vi "Increment_Variables_accel.vi"(0 "Accelerometer":waveform(dbl)[](array[waveform])=[{"t0"=timestamp(3695932468.9735494 s since 1904-01-01), "dt"=0.001015625, "Y"=[0.019294717668341704, 0.03864380419095477, -0.011709081788944725, -0.0416190732361809, -0.043655819185929645, -0.029323162502512563, 0.0026990099296482425, 0.0025104223417085417, -0.030530123065326632, -0.014575613125628141, 0.030044210180904515, 0.011411756492462309, 0.011675779115577892, 0.05037395216080402, 0.03887010929648241, 0.022802446804020104, -0.013368652562814068, -0.05123704022110553, -0.041053310472361805, -0.03415100475376884, -0.020120088211055275, 0.015221225768844215, 0.03291074151758794, 0.0006622639798994981, -0.04222255351758794, -0.05044497235175879, -0.047616158532663315, -0.03682894850251256, -0.026041738472361808, -0.006768086984924621, 0.0323072612361809, 0.03094943060301507, -0.006730369467336683, -0.035735140492462306, -0.017668449567839195, 0.016352751296482407, -0.005259386281407034, -0.021477918844221105, 0.014504592934673363, 0.056635060080402005, 0.050072212020100496, 0.04184979318592964, 0.019143847597989955, -0.009257443145728642, 0.02483919275376885, 0.0027744449648241173, 0.0039059704924623087, 0.03128888826130653, 0.0039059704924623087, 0.03498520498492462, 0.053579941155778896, 0.0218595088643216, 0.006923371899497488, 0.039511307095477385, 0.054334291507537685, 0.03419313711557789, 0.010996863798994977, -0.034226439788944726, -0.033094914261306535, -0.014651048160804023, 0.014165135276381913, 0.05599386228140703, 0.046300460261306534, 0.02921442479396985, -0.001638504592964822, -0.03852623679396985, -0.017479861979899494, 0.008620660190954775, -0.010464403708542715, -0.03618775070351758, -0.001336764452261309, 0.025442673035175875, -0.013481805115577887, 0.009450445577889446, 0.007753157286432159, -0.018007907226130652, 0.011223168904522615, -0.028908269809045224, -0.03950689225125628, -0.013180064974874374, 0.0145423104522613, 0.06338649572864322, 0.05252385066331658, 0.04656448288442211, 0.022576141698492466, -0.003147205296482415, 0.03698423341708543, 0.03860608667336683, -0.0006955666532663315, -0.022383139266331658, -0.0009595892763819072, 0.0520712404522613, 0.05931300382914573, 0.04928014415075377, 0.0396244596482412, 0.005112931055276382, 0.03434400718592964, 0.06602672195979899, 0.05060025726633166, 0.04909155656281407, 0.015070355698492466, 0.021482333688442212, 0.06904412336683417, 0.07209924229145728, 0.07074141165829145, 0.0710808693165829, 0.06851607812060301, 0.06723368252261307, 0.06557411174874371, 0.06157605488442211, 0.06199094757788945, 0.05633331993969849, 0.05210895796984924, 0.032873024, 0.008545225155778893, 0.04645133033165828, 0.06832749053266331, 0.05671049511557788, 0.05407026888442211, 0.04415056175879396, 0.015522965909547742, 0.007790874804020097, 0.05033623464321607, 0.052372980592964816, 0.032873024, 0.012203824361809043, -0.02445760273366834, -0.006692651949748746, 0.04177435815075377, 0.06640389713567839, 0.062179535165829136, 0.049883624432160795, 0.04286816616080402, 0.012694152090452257, -0.004844493587939695, 0.027932029195979896, 0.030232797768844216, -0.01687638169849246, -0.03818677913567839, -0.031322190934673366, -0.005561126422110554, 0.028384639407035173, 0.04520665225125628, 0.014881768110552765, -0.012689737246231153, 0.02189722638190955, -0.0015630695577889472, -0.004014708201005024, 0.01940787022110553, -0.01815877729648241, 0.009035552884422107, -0.0007710016884422133, -0.03158621355778894, 0.015786988532663318, 0.05365537619095477, 0.06059539942713567, 0.05033623464321607, 0.03977532971859296, 0.015862423567839193, -0.026192608542713568, -0.04233570607035175, -0.008616245346733671, -0.003034052743718596, -0.04576800017085427, -0.05161421539698492, -0.03550883538693467, -0.0341132872361809, 0.0026990099296482425, 0.026159305869346727, -0.0029586177085427143, 0.02246298914572864, 0.039322719507537685, -0.0004315440301507559, -0.03350980695477387, -0.033962417165829144, 0.003943688010050253, -0.013481805115577887, -0.0423734235879397, -0.03147306100502512, -0.009031138040201003, 0.03438172470351758, 0.05071340981909547, 0.025329520482412063, 0.001944659577889446, 0.04207609829145728, 0.05886039361809045, 0.041208595386934666, 0.03215639116582915, -0.007711024924623118, 0.020463960713567833, 0.025103215376884425, 0.006810219346733669, 0.05440972654271356, 0.06383910593969849, 0.055164076894472364, 0.04645133033165828, 0.03155291088442211, -0.006579499396984927, 0.0013788968140703503, 0.0176728644120603], "attributes"=variant("NI_ChannelName"=variant(string "cDAQ2Mod4/ai0"), "NI_UnitDescription"=variant(string "g"), "NI_dBReference"=variant(dbl 1.0))}, {"t0"=timestamp(3695932468.9735494 s since 1904-01-01), "dt"=0.001015625, "Y"=[0.009095719096509247, 0.02787151909650923, -0.02309687433264887, -0.05374730759753593, -0.056099101848049275, -0.04040762217659137, -0.008176474743326487, -0.00914032484599589, -0.04256664640657083, -0.027376368788501027, 0.019004098151950727, 0.0018475663244353208, 0.0016547963039014318, 0.04047867843942504, 0.026869114989733045, 0.010560771252566742, -0.024022170431211493, -0.06300026858316221, -0.05374730759753593, -0.045882290759753586, -0.03138598521560575, 0.003351172484599582, 0.02247395852156056, -0.010065620944558526, -0.0547497117043121, -0.06219063449691991, -0.05976173223819301, -0.04842685503080081, -0.03701486981519507, -0.01715955770020533, 0.022512512525667355, 0.020353488295687894, -0.016311369609856255, -0.04800276098562628, -0.02957394702258727, 0.006242722792607805, -0.018200515811088294, -0.03312091540041068, 0.003929482546201235, 0.04599190102669404, 0.039322058316221764, 0.03145704147843942, 0.007784882956878847, -0.02244145626283367, 0.014377617659137587, -0.007945150718685831, -0.0068656386036961, 0.02201131047227925, -0.006672868583162211, 0.024671536755646817, 0.04390998480492814, 0.012257147433264892, -0.004436736344969203, 0.029413679260780284, 0.04514371293634495, 0.02181854045174539, -0.00011868788501026573, -0.045419642710472274, -0.04511121067761806, -0.025911316632443532, 0.002040336344969196, 0.04595334702258727, 0.03673894004106776, 0.01861855811088295, -0.011723443121149896, -0.05023889322381929, -0.028532988911704305, -0.001429524024640652, -0.021747484188911703, -0.047617220944558517, -0.013458373305954827, 0.015418575770020537, -0.022749888295687887, -0.002393374127310055, -0.00451384435318275, -0.030267919096509235, -0.0005427819301848102, -0.039597988090349076, -0.05139551334702258, -0.025641438603696096, 0.003968036550308002, 0.0528545137577002, 0.04221360862422996, 0.0366618320328542, 0.011254743326488709, -0.014383669404517449, 0.027061885010266934, 0.028218505133470212, -0.012455969199178643, -0.03439319753593428, -0.01253307720739219, 0.04094132648870635, 0.04822803326488706, 0.03909073429158111, 0.029336571252566723, -0.005400586447638606, 0.024247442710472272, 0.05636292813141683, 0.04117265051334701, 0.03793411416837783, 0.004160806570841891, 0.011678837371663253, 0.059331586447638585, 0.06280144681724845, 0.061683380698151935, 0.061490610677618074, 0.058560506365503084, 0.05805930431211498, 0.05613160410677617, 0.051967771663244344, 0.05273885174537987, 0.04664731909650924, 0.04175096057494865, 0.022512512525667355, -0.0014680780287474327, 0.036199183983572886, 0.05925447843942505, 0.04830514127310062, 0.04417986283367556, 0.03307630965092401, 0.005008994661190966, -0.0022777121149897273, 0.03982326036960984, 0.04325456673511294, 0.023360700616016417, 0.0010764862422997928, -0.03578114168377823, -0.018547501848049278, 0.03126427145790553, 0.056594252156057484, 0.051389461601642705, 0.038936518275153986, 0.03323052566735113, 0.0014620262833675568, -0.017082449691991783, 0.019004098151950727, 0.020353488295687894, -0.027222152772073918, -0.0486196250513347, -0.04333772648870636, -0.016311369609856255, 0.018155910061601638, 0.035081117864476374, 0.003351172484599582, -0.024484818480492804, 0.011563175359342925, -0.012417415195071863, -0.014576439425051338, 0.008864395071868592, -0.02891852895277207, -0.0011981999999999965, -0.010952363039014368, -0.04179556632443532, 0.004623454620123202, 0.044218416837782326, 0.05250752772073922, 0.03966904435318275, 0.028719707186858318, 0.004315022587268999, -0.03759317987679671, -0.05316899753593428, -0.020012554004106772, -0.014268007392197121, -0.059800286242299786, -0.06488941478439425, -0.0461907227926078, -0.045419642710472274, -0.007212624640657084, 0.016652303901437376, -0.014113791375770013, 0.010830649281314164, 0.029220909240246395, -0.011260795071868585, -0.04507265667351129, -0.044802778644763855, -0.007945150718685831, -0.02413783244353182, -0.054055739630390134, -0.044648562628336746, -0.019742675975359336, 0.024864306776180706, 0.04229071663244352, 0.016305317864476393, -0.008060812731006159, 0.03191968952772073, 0.047341291170431204, 0.031302825462012324, 0.02247395852156056, -0.01904870390143737, 0.011177635318275148, 0.016305317864476393, -0.003241562217659144, 0.04452684887063654, 0.05485932197125257, 0.04595334702258727, 0.0365076160164271, 0.02181854045174539, -0.018046299794661186, -0.009988512936344965, 0.006088506776180697], "attributes"=variant("NI_ChannelName"=variant(string "cDAQ2Mod4/ai1"), "NI_UnitDescription"=variant(string "g"), "NI_dBReference"=variant(dbl 1.0))}, {"t0"=timestamp(3695932468.9735494 s since 1904-01-01), "dt"=0.001015625, "Y"=[0.02589708890303623, 0.04288576104799216, -0.00554298617042116, -0.03396775579823702, -0.036210848873653285, -0.02234779822722821, 0.008871644740450536, 0.008540696581782563, -0.023598046826640552, -0.00903632784524976, 0.035237181380999016, 0.01777047300685602, 0.017035032654260523, 0.05546179107737512, 0.04402569359451518, 0.02814018197845249, -0.005469442135161609, -0.04308721617042116, -0.03374712369245837, -0.02554696376101861, -0.013265109872673852, 0.02001356608227228, 0.038767295073457386, 0.008099432370225267, -0.034298703956905, -0.04367556845249755, -0.04091766713026445, -0.029408025612144957, -0.017898384094025468, 0.0018481893731635626, 0.03832603086190009, 0.03670806208619, 0.0012230650734573918, -0.029628657717923605, -0.011683913114593538, 0.022808239422135158, 0.0007450288442703186, -0.013963778207639572, 0.019682617923604307, 0.06009506529872673, 0.054946982830558266, 0.04637910272282075, 0.02299209951028403, -0.004954633888344762, 0.030898083300685598, 0.008834872722820759, 0.009202592899118508, 0.03648742998041135, 0.009717401145935351, 0.04016463174338883, 0.05689589976493632, 0.027404741625856998, 0.01302688273261508, 0.04520239815866796, 0.06009506529872673, 0.03784799463271302, 0.016667312477962774, -0.027091388501469152, -0.027091388501469152, -0.008227343457394714, 0.019204581694417234, 0.060646645563173354, 0.05167427326150831, 0.03468560111655239, 0.005856339294809009, -0.03098922237022527, -0.010727840656219395, 0.015159659755142014, -0.003998561429970619, -0.02870935727717924, 0.003429386131243873, 0.030567135142017626, -0.005726846258570034, 0.014718395543584718, 0.01302688273261508, -0.011794229167482862, 0.01637313633692458, -0.02227425419196866, -0.032386559040156714, -0.0074551310871694455, 0.019903250029382955, 0.06719206470127324, 0.05605014335945151, 0.05185813334965719, 0.028066637943192942, 0.0031719820078354513, 0.043437341312438774, 0.04317993718903035, 0.004091282448579821, -0.016243643300685603, 0.004348686571988242, 0.05538824704211556, 0.0630368267091087, 0.054064454407443674, 0.04428309771792359, 0.012364986415279135, 0.0403484918315377, 0.06994996602350635, 0.055866283271302636, 0.052740661772771785, 0.020932866523016642, 0.027625373731635646, 0.07399488796278157, 0.07822366999020566, 0.07495096042115572, 0.07590703287952986, 0.07333299164544563, 0.07248723523996081, 0.07112667058765915, 0.06579472803134181, 0.06612567619000978, 0.05958025705190988, 0.056270775465230155, 0.03884083910871694, 0.01519643177277179, 0.05075497282076395, 0.07322267559255631, 0.06307359872673848, 0.05814614836434867, 0.04917377606268364, 0.02148444678746327, 0.013799095102840348, 0.05590305528893241, 0.058109376346718894, 0.03946596340842311, 0.018653001429970614, -0.017346803829578848, -0.0006523078256611206, 0.047776439392752196, 0.07112667058765915, 0.06550055189030361, 0.05520438695396669, 0.048879599921645436, 0.01857945739471106, 0.0004140806856023464, 0.0333618084818805, 0.03630356989226248, -0.010360120479921648, -0.0313937145641528, -0.025399875690499514, 0.00045085270323211996, 0.034354652957884424, 0.051122692997061694, 0.022109571087169436, -0.005212038011753187, 0.028912394348677758, 0.005157670959843288, 0.002179137531831535, 0.02611772100881488, -0.011426508991185115, 0.015821556072477958, 0.0065550076297747235, -0.024076083055827622, 0.02291855547502448, 0.05950671301665034, 0.06605213215475024, 0.05472635072477962, 0.04428309771792359, 0.021337358716944168, -0.019038316640548485, -0.033820667727717926, -0.002490908707149856, 0.003907422360430946, -0.039704190548481885, -0.04632315372184133, -0.027532652713026448, -0.026797212360430953, 0.010158665357492647, 0.03225864795298726, 0.0012598370910871654, 0.02791954987267384, 0.04608492658178255, 0.006260831488736528, -0.026208860078354556, -0.025877911919686584, 0.01048961351616062, -0.005763618276199808, -0.03451933606268365, -0.023303870685602354, -0.0006890798432908941, 0.0388776111263467, 0.05616045941234084, 0.03317794839373163, 0.008540696581782563, 0.04593783851126346, 0.06255879047992163, 0.047371947198824677, 0.037553818491674815, -0.0025644527424094066, 0.0275518296963761, 0.03266314014691478, 0.013247514838393728, 0.06002152126346717, 0.06936161374142996, 0.06009506529872673, 0.05193167738491673, 0.037480274456415275, -2.71835259549498e-05, 0.007694940176297741, 0.022661151351616057], "attributes"=variant("NI_ChannelName"=variant(string "cDAQ2Mod4/ai2"), "NI_UnitDescription"=variant(string "g"), "NI_dBReference"=variant(dbl 1.0))}], 7 "Dummy Variable":dbl, 11 "error in 2":errorcluster) -> (1 "Y Accel Mag Array":dbl[](array[numeric])=[0.0033131967905544145, 0.011533831525713547, 0.008442061667059993, 0.009858654673222715, 0.008363300405539103, 0.002102550987145263, 0.004096487024183529, 0.00433165841994114, 0.00265508252937339, 0.005003543741433319, 0.0033674389332133095, 0.002412892363694339, 0.0017371897457633865, 0.0017333218339316864, 0.005254413350826224, 0.0073063809360835764, 0.00608380643471068, 0.0054542062991900335, 0.0023792094373612746, 0.004789200183006362, 0.007375237173938309, 0.003195183497815143, 0.0023576659519010824, 0.0031894685751027315, 0.0038472288041279876, 0.00184315376000046, 0.0050331931255288365, 0.0037747131768431563, 0.0014627035558359514, 0.003750056064901884, 0.005614898068157985, 0.005092169153670107, 0.006887608554409304, 0.0030983879127384735, 0.00214165531724511, 0.0003241083331647927, 0.0007980815831222994, 0.0035613760739590596, 0.00390793128896121, 0.003400370462350215, 0.004733205931244773, 0.003908201318260342, 0.000856924466573951, 0.0020338139877837543, 0.0026238508086522004, 0.000830066713475989, 0.0038902184256169644, 0.0031358154993883698, 0.0008589993939411568, 0.002873307167999069, 0.0023416434646463687, 0.0004510931593907119, 0.0004383783165562844, 0.0008874627311727322, 0.0012789681306284875, 0.0002755434129271385, 0.001522428187930964, 0.0025118502280273036, 0.0010763668998756048, 0.0017983248042534833, 0.0005603708597797223, 0.002488708057422721, 0.0034289499116928156, 0.0005141761317015294, 0.0005662749543606555, 0.0005895376750470246, 0.001316995707438423, 0.0019666607616864824, 0.0008909162596128791, 0.0018501545019689312, 0.0033674680981186198, 0.0018638646097661321, 0.0009231644052021042, 0.0013305685669963152, 0.00048467212646142815, 0.0010055563426380114, 0.0011922512362583773, 0.0013757679345206871, 0.001722787838392562, 0.001379941884811358, 0.0003961471539844812, 0.0017666790214067446, 0.0006913734583918143, 0.00154018788064677, 0.0010101793664572742, 0.00042212007045419495, 0.0006835355378316494, 0.001188644910899636, 0.00040022276319623824, 6.267596269438565e-05, 0.00011130714088648695, 0.00029044914834298766, 0.00013994679469761935, 9.599722391194053e-05, 0.00011490038035474606, 8.073681312813299e-05, 6.818183165259488e-05, 5.3847083164786216e-05, 4.243495671007987e-05, 3.670183062517156e-05], 3 "Y Accel Freq Array":dbl[](array[numeric])=[0.0, 4.923076923076923, 9.846153846153847, 14.76923076923077, 19.692307692307693, 24.615384615384617, 29.53846153846154, 34.46153846153847, 39.38461538461539, 44.30769230769231, 49.230769230769226, 54.153846153846146, 59.076923076923066, 63.999999999999986, 68.9230769230769, 73.84615384615383, 78.76923076923075, 83.69230769230766, 88.61538461538458, 93.5384615384615, 98.46153846153842, 103.38461538461534, 108.30769230769226, 113.23076923076918, 118.1538461538461, 123.07692307692302, 127.99999999999994, 132.92307692307688, 137.8461538461538, 142.76923076923075, 147.69230769230768, 152.6153846153846, 157.53846153846155, 162.46153846153848, 167.38461538461542, 172.30769230769235, 177.23076923076928, 182.15384615384622, 187.07692307692315, 192.00000000000009, 196.92307692307702, 201.84615384615395, 206.7692307692309, 211.69230769230782, 216.61538461538476, 221.5384615384617, 226.46153846153862, 231.38461538461556, 236.3076923076925, 241.23076923076943, 246.15384615384636, 251.0769230769233, 256.0000000000002, 260.92307692307713, 265.84615384615404, 270.76923076923094, 275.69230769230785, 280.61538461538476, 285.53846153846166, 290.46153846153857, 295.3846153846155, 300.3076923076924, 305.2307692307693, 310.1538461538462, 315.0769230769231, 320.0, 324.9230769230769, 329.8461538461538, 334.7692307692307, 339.6923076923076, 344.6153846153845, 349.53846153846143, 354.46153846153834, 359.38461538461524, 364.30769230769215, 369.23076923076906, 374.15384615384596, 379.07692307692287, 383.9999999999998, 388.9230769230767, 393.8461538461536, 398.7692307692305, 403.6923076923074, 408.6153846153843, 413.5384615384612, 418.4615384615381, 423.384615384615, 428.3076923076919, 433.23076923076883, 438.15384615384573, 443.07692307692264, 447.99999999999955, 452.92307692307645, 457.84615384615336, 462.76923076923026, 467.69230769230717, 472.6153846153841, 477.538461538461, 482.4615384615379, 487.3846153846148, 492.3076923076917, 497.2307692307686], 4 "Time Stamp":timestamp[](array[timestamp])=[timestamp(3695932468.9735494 s since 1904-01-01), timestamp(3695932468.974565 s since 1904-01-01), timestamp(3695932468.9755807 s since 1904-01-01), timestamp(3695932468.9765964 s since 1904-01-01), timestamp(3695932468.977612 s since 1904-01-01), timestamp(3695932468.9786277 s since 1904-01-01), timestamp(3695932468.9796433 s since 1904-01-01), timestamp(3695932468.980659 s since 1904-01-01), timestamp(3695932468.981674 s since 1904-01-01), timestamp(3695932468.98269 s since 1904-01-01), timestamp(3695932468.9837055 s since 1904-01-01), timestamp(3695932468.984721 s since 1904-01-01), timestamp(3695932468.985737 s since 1904-01-01), timestamp(3695932468.9867525 s since 1904-01-01), timestamp(3695932468.987768 s since 1904-01-01), timestamp(3695932468.988784 s since 1904-01-01), timestamp(3695932468.9897995 s since 1904-01-01), timestamp(3695932468.990815 s since 1904-01-01), timestamp(3695932468.991831 s since 1904-01-01), timestamp(3695932468.9928465 s since 1904-01-01), timestamp(3695932468.993862 s since 1904-01-01), timestamp(3695932468.9948773 s since 1904-01-01), timestamp(3695932468.995893 s since 1904-01-01), timestamp(3695932468.9969087 s since 1904-01-01), timestamp(3695932468.9979243 s since 1904-01-01), timestamp(3695932468.99894 s since 1904-01-01), timestamp(3695932468.9999557 s since 1904-01-01), timestamp(3695932469.0009713 s since 1904-01-01), timestamp(3695932469.001987 s since 1904-01-01), timestamp(3695932469.0030026 s since 1904-01-01), timestamp(3695932469.0040183 s since 1904-01-01), timestamp(3695932469.005034 s since 1904-01-01), timestamp(3695932469.0060496 s since 1904-01-01), timestamp(3695932469.007065 s since 1904-01-01), timestamp(3695932469.0080805 s since 1904-01-01), timestamp(3695932469.009096 s since 1904-01-01), timestamp(3695932469.010112 s since 1904-01-01), timestamp(3695932469.0111275 s since 1904-01-01), timestamp(3695932469.012143 s since 1904-01-01), timestamp(3695932469.013159 s since 1904-01-01), timestamp(3695932469.0141745 s since 1904-01-01), timestamp(3695932469.01519 s since 1904-01-01), timestamp(3695932469.016206 s since 1904-01-01), timestamp(3695932469.0172215 s since 1904-01-01), timestamp(3695932469.018237 s since 1904-01-01), timestamp(3695932469.019253 s since 1904-01-01), timestamp(3695932469.020268 s since 1904-01-01), timestamp(3695932469.0212836 s since 1904-01-01), timestamp(3695932469.0222993 s since 1904-01-01), timestamp(3695932469.023315 s since 1904-01-01), timestamp(3695932469.0243306 s since 1904-01-01), timestamp(3695932469.0253463 s since 1904-01-01), timestamp(3695932469.026362 s since 1904-01-01), timestamp(3695932469.0273776 s since 1904-01-01), timestamp(3695932469.0283933 s since 1904-01-01), timestamp(3695932469.029409 s since 1904-01-01), timestamp(3695932469.0304246 s since 1904-01-01), timestamp(3695932469.0314403 s since 1904-01-01), timestamp(3695932469.0324554 s since 1904-01-01), timestamp(3695932469.033471 s since 1904-01-01), timestamp(3695932469.034487 s since 1904-01-01), timestamp(3695932469.0355024 s since 1904-01-01), timestamp(3695932469.036518 s since 1904-01-01), timestamp(3695932469.0375338 s since 1904-01-01), timestamp(3695932469.0385494 s since 1904-01-01), timestamp(3695932469.039565 s since 1904-01-01), timestamp(3695932469.0405807 s since 1904-01-01), timestamp(3695932469.0415964 s since 1904-01-01), timestamp(3695932469.042612 s since 1904-01-01), timestamp(3695932469.0436277 s since 1904-01-01), timestamp(3695932469.0446434 s since 1904-01-01), timestamp(3695932469.0456586 s since 1904-01-01), timestamp(3695932469.0466743 s since 1904-01-01), timestamp(3695932469.04769 s since 1904-01-01), timestamp(3695932469.0487056 s since 1904-01-01), timestamp(3695932469.0497212 s since 1904-01-01), timestamp(3695932469.050737 s since 1904-01-01), timestamp(3695932469.0517526 s since 1904-01-01), timestamp(3695932469.052768 s since 1904-01-01), timestamp(3695932469.053784 s since 1904-01-01), timestamp(3695932469.0547996 s since 1904-01-01), timestamp(3695932469.055815 s since 1904-01-01), timestamp(3695932469.056831 s since 1904-01-01), timestamp(3695932469.057846 s since 1904-01-01), timestamp(3695932469.0588617 s since 1904-01-01), timestamp(3695932469.0598774 s since 1904-01-01), timestamp(3695932469.060893 s since 1904-01-01), timestamp(3695932469.0619087 s since 1904-01-01), timestamp(3695932469.0629244 s since 1904-01-01), timestamp(3695932469.06394 s since 1904-01-01), timestamp(3695932469.0649557 s since 1904-01-01), timestamp(3695932469.0659714 s since 1904-01-01), timestamp(3695932469.066987 s since 1904-01-01), timestamp(3695932469.0680027 s since 1904-01-01), timestamp(3695932469.0690184 s since 1904-01-01), timestamp(3695932469.070034 s since 1904-01-01), timestamp(3695932469.071049 s since 1904-01-01), timestamp(3695932469.072065 s since 1904-01-01), timestamp(3695932469.0730805 s since 1904-01-01), timestamp(3695932469.074096 s since 1904-01-01), timestamp(3695932469.075112 s since 1904-01-01), timestamp(3695932469.0761275 s since 1904-01-01), timestamp(3695932469.077143 s since 1904-01-01), timestamp(3695932469.078159 s since 1904-01-01), timestamp(3695932469.0791745 s since 1904-01-01), timestamp(3695932469.08019 s since 1904-01-01), timestamp(3695932469.081206 s since 1904-01-01), timestamp(3695932469.0822215 s since 1904-01-01), timestamp(3695932469.0832367 s since 1904-01-01), timestamp(3695932469.0842524 s since 1904-01-01), timestamp(3695932469.085268 s since 1904-01-01), timestamp(3695932469.0862837 s since 1904-01-01), timestamp(3695932469.0872993 s since 1904-01-01), timestamp(3695932469.088315 s since 1904-01-01), timestamp(3695932469.0893307 s since 1904-01-01), timestamp(3695932469.0903463 s since 1904-01-01), timestamp(3695932469.091362 s since 1904-01-01), timestamp(3695932469.0923777 s since 1904-01-01), timestamp(3695932469.0933933 s since 1904-01-01), timestamp(3695932469.094409 s since 1904-01-01), timestamp(3695932469.0954247 s since 1904-01-01), timestamp(3695932469.09644 s since 1904-01-01), timestamp(3695932469.0974555 s since 1904-01-01), timestamp(3695932469.098471 s since 1904-01-01), timestamp(3695932469.099487 s since 1904-01-01), timestamp(3695932469.1005025 s since 1904-01-01), timestamp(3695932469.101518 s since 1904-01-01), timestamp(3695932469.102534 s since 1904-01-01), timestamp(3695932469.1035495 s since 1904-01-01), timestamp(3695932469.104565 s since 1904-01-01), timestamp(3695932469.105581 s since 1904-01-01), timestamp(3695932469.1065965 s since 1904-01-01), timestamp(3695932469.107612 s since 1904-01-01), timestamp(3695932469.1086273 s since 1904-01-01), timestamp(3695932469.109643 s since 1904-01-01), timestamp(3695932469.1106586 s since 1904-01-01), timestamp(3695932469.1116743 s since 1904-01-01), timestamp(3695932469.11269 s since 1904-01-01), timestamp(3695932469.1137056 s since 1904-01-01), timestamp(3695932469.1147213 s since 1904-01-01), timestamp(3695932469.115737 s since 1904-01-01), timestamp(3695932469.1167526 s since 1904-01-01), timestamp(3695932469.1177683 s since 1904-01-01), timestamp(3695932469.118784 s since 1904-01-01), timestamp(3695932469.1197996 s since 1904-01-01), timestamp(3695932469.1208153 s since 1904-01-01), timestamp(3695932469.1218305 s since 1904-01-01), timestamp(3695932469.122846 s since 1904-01-01), timestamp(3695932469.123862 s since 1904-01-01), timestamp(3695932469.1248775 s since 1904-01-01), timestamp(3695932469.125893 s since 1904-01-01), timestamp(3695932469.126909 s since 1904-01-01), timestamp(3695932469.1279244 s since 1904-01-01), timestamp(3695932469.12894 s since 1904-01-01), timestamp(3695932469.129956 s since 1904-01-01), timestamp(3695932469.1309714 s since 1904-01-01), timestamp(3695932469.131987 s since 1904-01-01), timestamp(3695932469.1330028 s since 1904-01-01), timestamp(3695932469.134018 s since 1904-01-01), timestamp(3695932469.1350336 s since 1904-01-01), timestamp(3695932469.1360493 s since 1904-01-01), timestamp(3695932469.137065 s since 1904-01-01), timestamp(3695932469.1380806 s since 1904-01-01), timestamp(3695932469.1390963 s since 1904-01-01), timestamp(3695932469.140112 s since 1904-01-01), timestamp(3695932469.1411276 s since 1904-01-01), timestamp(3695932469.1421432 s since 1904-01-01), timestamp(3695932469.143159 s since 1904-01-01), timestamp(3695932469.1441746 s since 1904-01-01), timestamp(3695932469.1451902 s since 1904-01-01), timestamp(3695932469.146206 s since 1904-01-01), timestamp(3695932469.147221 s since 1904-01-01), timestamp(3695932469.1482368 s since 1904-01-01), timestamp(3695932469.1492524 s since 1904-01-01), timestamp(3695932469.150268 s since 1904-01-01), timestamp(3695932469.1512837 s since 1904-01-01), timestamp(3695932469.1522994 s since 1904-01-01), timestamp(3695932469.153315 s since 1904-01-01), timestamp(3695932469.1543307 s since 1904-01-01), timestamp(3695932469.1553464 s since 1904-01-01), timestamp(3695932469.156362 s since 1904-01-01), timestamp(3695932469.1573777 s since 1904-01-01), timestamp(3695932469.1583934 s since 1904-01-01), timestamp(3695932469.1594086 s since 1904-01-01), timestamp(3695932469.160424 s since 1904-01-01), timestamp(3695932469.16144 s since 1904-01-01), timestamp(3695932469.1624556 s since 1904-01-01), timestamp(3695932469.163471 s since 1904-01-01), timestamp(3695932469.164487 s since 1904-01-01), timestamp(3695932469.1655025 s since 1904-01-01), timestamp(3695932469.166518 s since 1904-01-01), timestamp(3695932469.167534 s since 1904-01-01), timestamp(3695932469.1685495 s since 1904-01-01), timestamp(3695932469.169565 s since 1904-01-01), timestamp(3695932469.170581 s since 1904-01-01), timestamp(3695932469.1715965 s since 1904-01-01), timestamp(3695932469.1726117 s since 1904-01-01), timestamp(3695932469.1736274 s since 1904-01-01), timestamp(3695932469.174643 s since 1904-01-01), timestamp(3695932469.1756587 s since 1904-01-01)], 6 "Dummy Variable Array":dbl[](array[numeric]), 9 "Z Accel Mag Array":dbl[](array[numeric])=[0.019971462122086184, 0.010948382379644262, 0.008116146087008579, 0.009333779096660784, 0.007905689922427317, 0.0020141279435321657, 0.003907476661038542, 0.0040954659603004125, 0.0024616831066559372, 0.004927802212947944, 0.0031728006052821616, 0.002272476268580278, 0.0016080610335601623, 0.0015579207225638976, 0.0049624358972122536, 0.0070204493778668765, 0.0058592603641987335, 0.005259479474125528, 0.0023367638475221366, 0.0045880301585258885, 0.007052524044945366, 0.0029363813126921127, 0.0021923520752701237, 0.0030988387898563934, 0.003642690710579167, 0.0018027234552405397, 0.004898683929895741, 0.003691348825521774, 0.0014684640929464065, 0.003585471062261296, 0.005378721500984641, 0.004769939578854797, 0.006598046597686076, 0.0029367202322358424, 0.0019460970143305135, 0.00035413950904622326, 0.0008295409097351278, 0.003325350799986514, 0.00377242558359643, 0.0032074040330492834, 0.004426589992784921, 0.003794697139499976, 0.0008052303514485751, 0.001914695306719483, 0.00254743200188537, 0.0007544983066559986, 0.003790949329882019, 0.003050902230848892, 0.0006803812768082399, 0.0027088434549860075, 0.0022633501703134386, 0.00033034885621119814, 0.0004036772578109767, 0.0008640752596650803, 0.0011349160628484557, 0.0003749189898309628, 0.001558374918616446, 0.0024724480295184796, 0.0010730890325214271, 0.0016961991425869908, 0.00045795013745203553, 0.0024226249041348065, 0.0032532231481419817, 0.0004129710275067112, 0.0005696272336993551, 0.0005611040476604964, 0.0012619731212988212, 0.0018756463869423364, 0.0008514530419130162, 0.001761934357230495, 0.0032391497407567695, 0.0019089808499032747, 0.0009772329871434223, 0.0012370104429501507, 0.0005321822329501325, 0.0009609983634478406, 0.0011826039630110545, 0.0013560728290809166, 0.0016305703597276635, 0.0013218903473141128, 0.00042751616219297137, 0.0017702317973107297, 0.00056973355370719, 0.00153288910785441, 0.0008956914805150511, 0.0004125033113066504, 0.0006629875325086497, 0.0011410141811447443, 0.0004012827212918755, 8.469052368293879e-05, 0.00010391150477690947, 0.0002759738462935365, 0.0001323075454136867, 8.357451095835174e-05, 0.0001046663491791139, 7.264792717025675e-05, 6.0884155482983634e-05, 4.859446359026642e-05, 3.834811261419187e-05, 3.147710182830082e-05], 10 "X Accel Freq Array":dbl[](array[numeric])=[0.0, 4.923076923076923, 9.846153846153847, 14.76923076923077, 19.692307692307693, 24.615384615384617, 29.53846153846154, 34.46153846153847, 39.38461538461539, 44.30769230769231, 49.230769230769226, 54.153846153846146, 59.076923076923066, 63.999999999999986, 68.9230769230769, 73.84615384615383, 78.76923076923075, 83.69230769230766, 88.61538461538458, 93.5384615384615, 98.46153846153842, 103.38461538461534, 108.30769230769226, 113.23076923076918, 118.1538461538461, 123.07692307692302, 127.99999999999994, 132.92307692307688, 137.8461538461538, 142.76923076923075, 147.69230769230768, 152.6153846153846, 157.53846153846155, 162.46153846153848, 167.38461538461542, 172.30769230769235, 177.23076923076928, 182.15384615384622, 187.07692307692315, 192.00000000000009, 196.92307692307702, 201.84615384615395, 206.7692307692309, 211.69230769230782, 216.61538461538476, 221.5384615384617, 226.46153846153862, 231.38461538461556, 236.3076923076925, 241.23076923076943, 246.15384615384636, 251.0769230769233, 256.0000000000002, 260.92307692307713, 265.84615384615404, 270.76923076923094, 275.69230769230785, 280.61538461538476, 285.53846153846166, 290.46153846153857, 295.3846153846155, 300.3076923076924, 305.2307692307693, 310.1538461538462, 315.0769230769231, 320.0, 324.9230769230769, 329.8461538461538, 334.7692307692307, 339.6923076923076, 344.6153846153845, 349.53846153846143, 354.46153846153834, 359.38461538461524, 364.30769230769215, 369.23076923076906, 374.15384615384596, 379.07692307692287, 383.9999999999998, 388.9230769230767, 393.8461538461536, 398.7692307692305, 403.6923076923074, 408.6153846153843, 413.5384615384612, 418.4615384615381, 423.384615384615, 428.3076923076919, 433.23076923076883, 438.15384615384573, 443.07692307692264, 447.99999999999955, 452.92307692307645, 457.84615384615336, 462.76923076923026, 467.69230769230717, 472.6153846153841, 477.538461538461, 482.4615384615379, 487.3846153846148, 492.3076923076917, 497.2307692307686], 12 "Z Accel Freq Array":dbl[](array[numeric])=[0.0, 4.923076923076923, 9.846153846153847, 14.76923076923077, 19.692307692307693, 24.615384615384617, 29.53846153846154, 34.46153846153847, 39.38461538461539, 44.30769230769231, 49.230769230769226, 54.153846153846146, 59.076923076923066, 63.999999999999986, 68.9230769230769, 73.84615384615383, 78.76923076923075, 83.69230769230766, 88.61538461538458, 93.5384615384615, 98.46153846153842, 103.38461538461534, 108.30769230769226, 113.23076923076918, 118.1538461538461, 123.07692307692302, 127.99999999999994, 132.92307692307688, 137.8461538461538, 142.76923076923075, 147.69230769230768, 152.6153846153846, 157.53846153846155, 162.46153846153848, 167.38461538461542, 172.30769230769235, 177.23076923076928, 182.15384615384622, 187.07692307692315, 192.00000000000009, 196.92307692307702, 201.84615384615395, 206.7692307692309, 211.69230769230782, 216.61538461538476, 221.5384615384617, 226.46153846153862, 231.38461538461556, 236.3076923076925, 241.23076923076943, 246.15384615384636, 251.0769230769233, 256.0000000000002, 260.92307692307713, 265.84615384615404, 270.76923076923094, 275.69230769230785, 280.61538461538476, 285.53846153846166, 290.46153846153857, 295.3846153846155, 300.3076923076924, 305.2307692307693, 310.1538461538462, 315.0769230769231, 320.0, 324.9230769230769, 329.8461538461538, 334.7692307692307, 339.6923076923076, 344.6153846153845, 349.53846153846143, 354.46153846153834, 359.38461538461524, 364.30769230769215, 369.23076923076906, 374.15384615384596, 379.07692307692287, 383.9999999999998, 388.9230769230767, 393.8461538461536, 398.7692307692305, 403.6923076923074, 408.6153846153843, 413.5384615384612, 418.4615384615381, 423.384615384615, 428.3076923076919, 433.23076923076883, 438.15384615384573, 443.07692307692264, 447.99999999999955, 452.92307692307645, 457.84615384615336, 462.76923076923026, 467.69230769230717, 472.6153846153841, 477.538461538461, 482.4615384615379, 487.3846153846148, 492.3076923076917, 497.2307692307686], 14 "X Accel Mag Array":dbl[](array[numeric])=[0.014040667468341707, 0.011305846455333925, 0.008293929195544896, 0.009560383109368591, 0.008179581864891134, 0.0019285003887053891, 0.0039802820206588, 0.004262296856518639, 0.00264036033635322, 0.00495567381828343, 0.00324381068066818, 0.002210578802966312, 0.0016004770983194625, 0.0016417712329695896, 0.005154974925259235, 0.007251271540632396, 0.005970472935431034, 0.0053193452140212595, 0.002344027870445127, 0.004639864150921315, 0.0072439910411350415, 0.0031400095410323544, 0.0022820268295372123, 0.0031270695618889083, 0.0037307768041843796, 0.0017171069127818591, 0.004982205632497811, 0.003874058144300419, 0.0015743617625346466, 0.003728787703377941, 0.005518740054984088, 0.004932839517027118, 0.006736951958719054, 0.0030808214145690753, 0.002094167093990494, 0.000290018834947526, 0.0008583155497920036, 0.0034858449316966266, 0.0038047332169444032, 0.0033299396101555494, 0.004532174238939295, 0.0038004864657253494, 0.0008222454805304883, 0.001987448220344883, 0.002533470967294649, 0.00079897975532402, 0.0038232479485662205, 0.0031219666486457004, 0.0008567684154450162, 0.0028473811132765843, 0.002356089789119549, 0.0004111229614004419, 0.00041955022117880214, 0.0008533688490751977, 0.0011673217322755646, 0.0003079441848912749, 0.0014898244758079712, 0.0025350489499428716, 0.001156536583870256, 0.0017003400631796432, 0.0005160883022773624, 0.002482478901245743, 0.0032601434978507936, 0.0003672945856646527, 0.0005146735244742892, 0.0005241824949543067, 0.0011201884809814296, 0.001961411508547202, 0.0008650361134341148, 0.0018823693611651812, 0.0033648500365931295, 0.0018641018132155179, 0.0009302178222994041, 0.001248444592007628, 0.0004270421935762477, 0.0011182974398200774, 0.0012369383465182676, 0.001430905833430144, 0.0017319388019678555, 0.001354191220596254, 0.0004549424155323687, 0.0017023835212825026, 0.0005401123374231916, 0.0014494579152306711, 0.0010012351197536168, 0.000391078887312264, 0.0007372295547393363, 0.001199537329360829, 0.0003739987963654897, 5.988527957018166e-05, 0.00010386824549758468, 0.0002879288715795099, 0.00013372976332235516, 9.697771818388118e-05, 0.0001152943308889597, 8.06219099249761e-05, 7.311040932559463e-05, 6.0259574236751743e-05, 5.3026690698572274e-05, 4.72977578646794e-05], 15 "error IO":errorcluster)   [LabVIEW 2016]
uses:
  <vilib>/Utility/error.llb/DialogType.ctl
  <vilib>/express/express analysis/Spectral/Block/exnSpectralBlock spectral measurements RMS poly.vi
  <vilib>/express/express analysis/Spectral/Block/exnSpectralBlock spectral measurements RMS array WFM.vi
  <vilib>/express/express analysis/Spectral/XNode/ExpressSpectralMeasurementsBlockNode.xnode
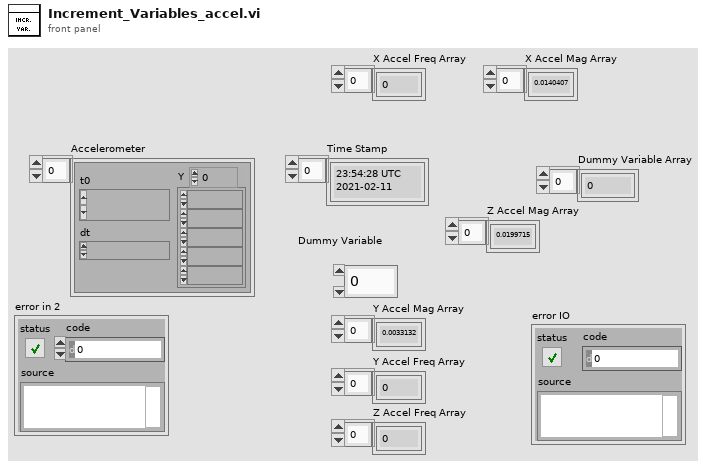
[diagram p1: front panel]
types:
  T1 = cluster{"averaging mode":u16, "weighting mode":u16, "number of averages":u32}
  T2 = cluster{"dB On (F)":bool, "unwrap phase (F)":bool, "convert to degree (F)":bool}
  T3 = typedef "DialogType.ctl" = u16
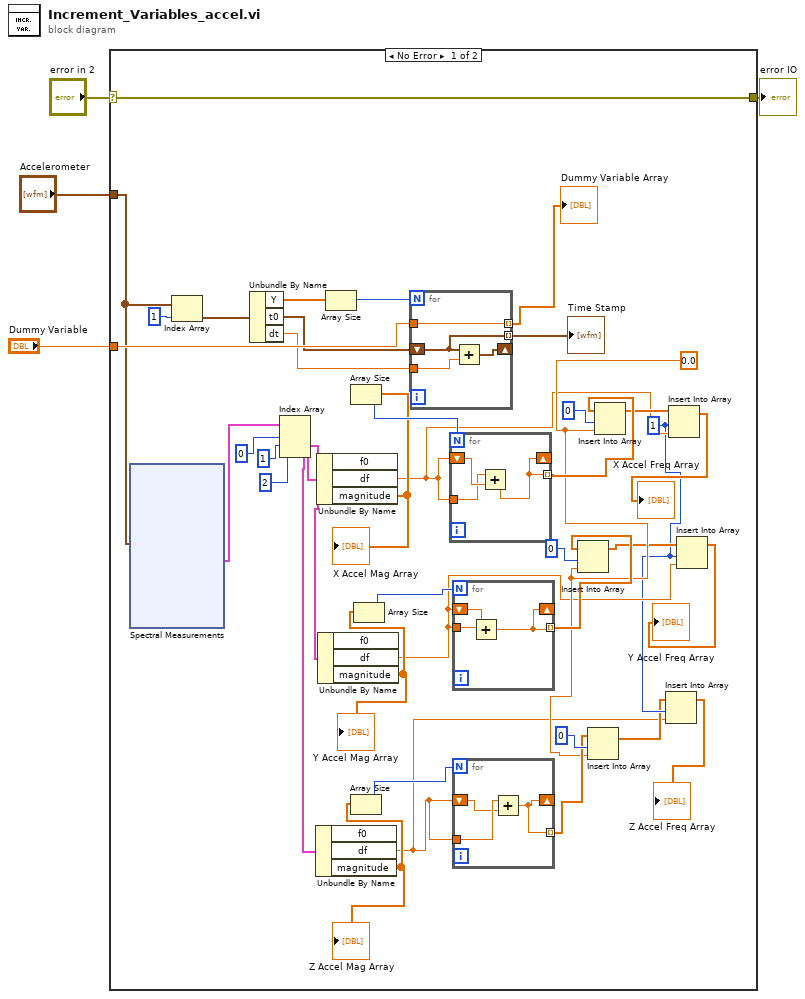
[diagram p0: block diagram]
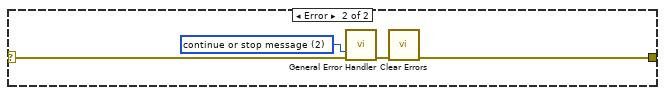
[diagram p2: hidden frame]
diagram:
  n1 = case shown="No Error" "error in 2" {
    selector: "error in 2" -> [w38 w70]
    tunnel: "Dummy Variable" -> [w45 _]
    tunnel: "Accelerometer" -> [w35 _]
    tunnel: [w38 w69] -> w2
    frame No Error {
      w8 = 1 ("index")
      w15 = 0.0 ("new element/subarray")
      n2 = xnode "Spectral Measurements"("Signals"=w35) -> ("FFT - (RMS)"=w34:cluster{"f0":dbl, "df":dbl, "magnitude":dbl[]}[])  [unwired: 1 in, 2 out]
      n3 = Index Array(array=w35, index=1) -> (element=w43:waveform(dbl))
      n4 = Unbundle By Name(w43) -> ("Y"=w39:dbl[], "t0"=w41:timestamp, "dt"=w42:dbl)
      n5 = Index Array(array=w34, index #1=0 ("index"), index #2=1 ("index"), index #3=2 ("index")) -> (element #1=w32:cluster{"f0":dbl, "df":dbl, "magnitude":dbl[]}, element #2=w27:cluster{"f0":dbl, "df":dbl, "magnitude":dbl[]}, element #3=w26:cluster{"f0":dbl, "df":dbl, "magnitude":dbl[]})
      n6 = Unbundle By Name(w26) -> ("df"=w6:dbl, "magnitude"=w22:dbl[])  [unwired: 1 out]
      "Z Accel Mag Array" <- w22
      n7 = Unbundle By Name(w32) -> ("df"=w13:dbl, "magnitude"=w30:dbl[])  [unwired: 1 out]
      "X Accel Mag Array" <- w30
      n8 = Unbundle By Name(w27) -> ("df"=w10:dbl, "magnitude"=w24:dbl[])  [unwired: 1 out]
      "Y Accel Mag Array" <- w24
      n9 = Array Size(array=w39) -> (size(s)=w40:i32)
      n10 = Array Size(array=w30) -> (size(s)=w31:i32)
      n11 = Array Size(array=w22) -> (size(s)=w23:i32)
      n12 = Array Size(array=w24) -> (size(s)=w25:i32)
      n13 = for {
        N: w40 -> [_]
        tunnel: w42 -> [w68]
        shift-right: [w67] -> _
        shift-left: w41 -> [w66]
        tunnel: [w66] -> w36 mode=indexing
        tunnel: [w65] -> w37 mode=indexing
        tunnel: w45 -> [w65]
        n14 = Add(x=w66, y=w68) -> (x+y=w67:timestamp)
      }
      "Time Stamp" <- w36
      "Dummy Variable Array" <- w37
      n15 = for {
        N: w31 -> [_]
        shift-right: [w52] -> _
        shift-left: w13 -> [w54]
        tunnel: w13 -> [w53]
        tunnel: [w52] -> w20 mode=indexing
        n16 = Add(x=w53, y=w54) -> (x+y=w52:dbl)
      }
      n17 = for {
        N: w25 -> [_]
        tunnel: [w49] -> w18 mode=indexing
        shift-right: [w49] -> _
        shift-left: w10 -> [w50]
        tunnel: w10 -> [w51]
        n18 = Add(x=w51, y=w50) -> (x+y=w49:dbl)
      }
      n19 = for {
        N: w23 -> [_]
        tunnel: w6 -> [w48]
        shift-right: [w46] -> _
        shift-left: w6 -> [w47]
        tunnel: [w46] -> w16 mode=indexing
        n20 = Add(x=w48, y=w47) -> (x+y=w46:dbl)
      }
      n21 = Insert Into Array(array=w18, index=0, new element=w15) -> (w11:dbl[])
      n22 = Insert Into Array(array=w16, index=0, new element=w15) -> (w7:dbl[])
      n23 = Insert Into Array(array=w20, index=0, new element=w15) -> (w14:dbl[])
      n24 = Insert Into Array(array=w7, index=w8, new element=w6) -> (→"Z Accel Freq Array":dbl[])
      n25 = Insert Into Array(array=w14, index=w8, new element=w13) -> (→"X Accel Freq Array":dbl[])
      n26 = Insert Into Array(array=w11, index=w8, new element=w10) -> (→"Y Accel Freq Array":dbl[])
    }
    frame Error {
      w71 = T3 2 items=["no dialog", "OK message", "continue or stop message", "OK message + warnings", "continue/stop + warnings"] ("type of dialog (OK msg:1)")
      n27 = call <vilib>:"General Error Handler.vi"("type of dialog (OK msg:1)"=w71, "error in (no error)"=w70) -> ("error out"=w72:errorcluster)  [unwired: 9 in, 4 out]
      n28 = call <vilib>:"Clear Errors.vi"("error in (no error)"=w72) -> ("error out"=w69:errorcluster)  [unwired: 5 in, 1 out]
    }
  }
  "error IO" <- w2
